vi "find method.vi"(8 "error in (no error)":errorcluster, 10 "String":string, 11 "Variant":variant) -> (0 "error out":errorcluster, 2 "Boolean":bool, 3 "VI out":refnum<vi>)   [LabVIEW 2017]
uses:
  <vilib>/NI/JSON Support for LabVIEW/JSON Value/JSON Value.lvclass
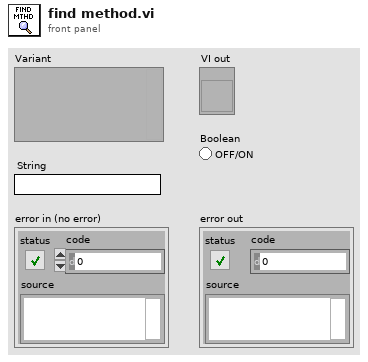
[diagram p1: front panel]
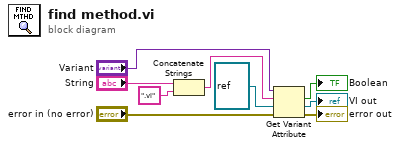
[diagram p0: block diagram]
diagram:
  n1 = Concatenate Strings("String", ".vi" ("string")) -> (w9:string)
  n2 = Get Variant Attribute(Variant="Variant", name=w9, default value (empty Variant)=refnum<vi> refnum ("type specifier VI Refnum (for type only)"), error in="error in (no error)") -> (found=→"Boolean":bool, value=→"VI out":refnum<vi>, error out=→"error out":errorcluster)  [unwired: 1 out]
